vi "VPA QC Choose Printer.vi"() -> (2 "Cancelled":bool)   [LabVIEW 2013]
panel:
  in  "Cancel":bool
  in  "Print":bool
  in  "Choose a Printer":u16(ring) items=["Microsoft XPS Document Writer", "Bullzip PDF Printer", "Auto HP DeskJet 1220C on NEWXPOFFICE", "Auto Canon MF4100 Series UFRII LT on NEWXPOFFICE", "\\\\newxpoffice\\Canon MF4100 Series UFRII LT"]
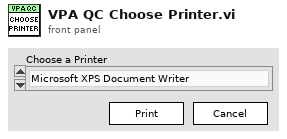
[diagram p1: front panel]
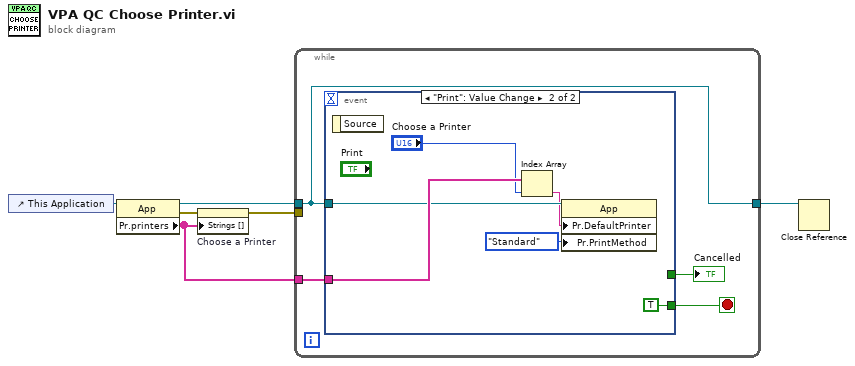
[diagram p0: block diagram]
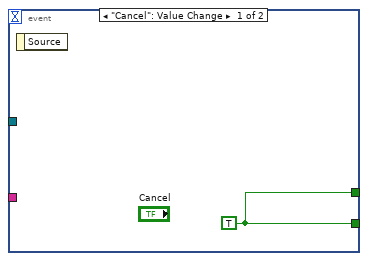
[diagram p2: hidden frame]
diagram:
  n1 = control-ref of="This Application"() -> (w6:refnum<vi>)
  n2 = property class="App"(reference=w6) -> (reference out=w3:refnum<vi>, error out=w5:errorcluster, "Pr.printers"=w2:string[])  [unwired: 1 in]
  n3 = property on="Choose a Printer" class="Ring (strict)"(error in=w5, "Strings []"=w2) -> (error out=w4:errorcluster)  [unwired: 1 in, 1 out]
  n4 = while {
    tunnel: w4 -> [_]
    tunnel: w3 -> [w7]
    tunnel: w2 -> [w8]
    tunnel: [w7] -> w1
    stop <- w10 stop-if-true
    n5 = event shown="[1] \"Print\": Value Change" {
      selector: _ -> [_ _]
      dyn-events: _ -> [_ _]
      timeout: _ -> [_ _]
      tunnel: [w11 TRUE] -> w10
      tunnel: [w11 _] -> w9
      tunnel: w7 -> [_ w14]
      tunnel: w8 -> [_ w16]
      event "Cancel": Value Change {
        w11 = TRUE
        n6 = event-data() -> ()  [unwired: 1 in, 1 out]
      }
      event "Print": Value Change {
        n7 = event-data() -> ()  [unwired: 1 in, 1 out]
        n8 = Index Array(array=w16, index="Choose a Printer") -> (element=w13:string)
        n9 = property class="App"(reference=w14, "Pr.DefaultPrinter"=w13, "Pr.PrintMethod"=enum32{"Standard", "PostScript", "Bitmap"}."Standard" ("Printing:Method")) -> ()  [unwired: 1 in, 2 out]
      }
    }
    "Cancelled" <- w9
  }
  n10 = Close Reference(reference=w1) -> ()  [unwired: 1 in, 1 out]
